vi "mod_Create Continuous MSK.vi"(0 "PN Sequence Order":i32, 1 "MSK System Parameters":T2, 3 "TX Filter":T1(ring), 4 "Filter Length":i32, 5 "error in (no error)":errorcluster, 6 "Symbol Rate, Hz":dbl format="%.2f", 7 "Alpha":dbl format="%.2f") -> (14 "output complex waveform":T3 {"Y" format="%.3f"; "dt" format="%^.2e"; "t0" format="%.4f"}, 17 "samples per symbol":i32, 19 "error out":errorcluster)   [LabVIEW 2020, in "niDMT.lvlib"]
uses:
  <vilib>/addons/Modulation/niDMT.lvlib
  <vilib>/addons/Modulation/Analog/controls/Complex Data Waveform.ctl
  <vilib>/addons/Modulation/Digital/Support/Controls/MSK System Parameters.ctl
  <vilib>/addons/Modulation/Digital/General/MT Generate Bits (Galois, PN Order).vi
  <vilib>/addons/Modulation/Analog/support/mod_Set Error Source.vi
  <vilib>/addons/Modulation/Digital/Support/Common/Validators/mod_Generate Bits Validate.vi
  <vilib>/addons/Modulation/Digital/Support/Common/Validators/mod_Generate Filter Coefficients Validate.vi
  <vilib>/addons/Modulation/Digital/General/subVIs/mod_Generate Filter Coefficients.vi
  <vilib>/addons/Modulation/Digital/General/subVIs/mod_Generate Bits PN Sequence.vi
  <vilib>/addons/Modulation/niAMT.lvlib
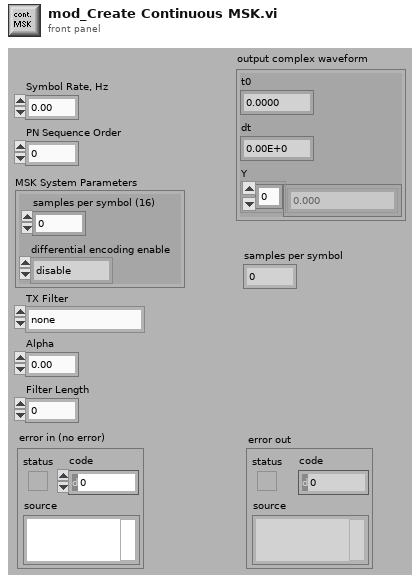
[diagram p1: front panel]
types:
  T1 = enum16{"none", "Raised Cosine", "Root Raised Cos", "Gaussian"}
  T2 = typedef "niDMT.lvlib/MSK System Parameters.ctl" = cluster{"differential encoding enable":enum16{"disable", "enable"}, "samples per symbol (16)":i32}
  T3 = typedef "niAMT.lvlib/Complex Data Waveform.ctl" = cluster{"t0":dbl, "dt":dbl, "Y":cdb[]}
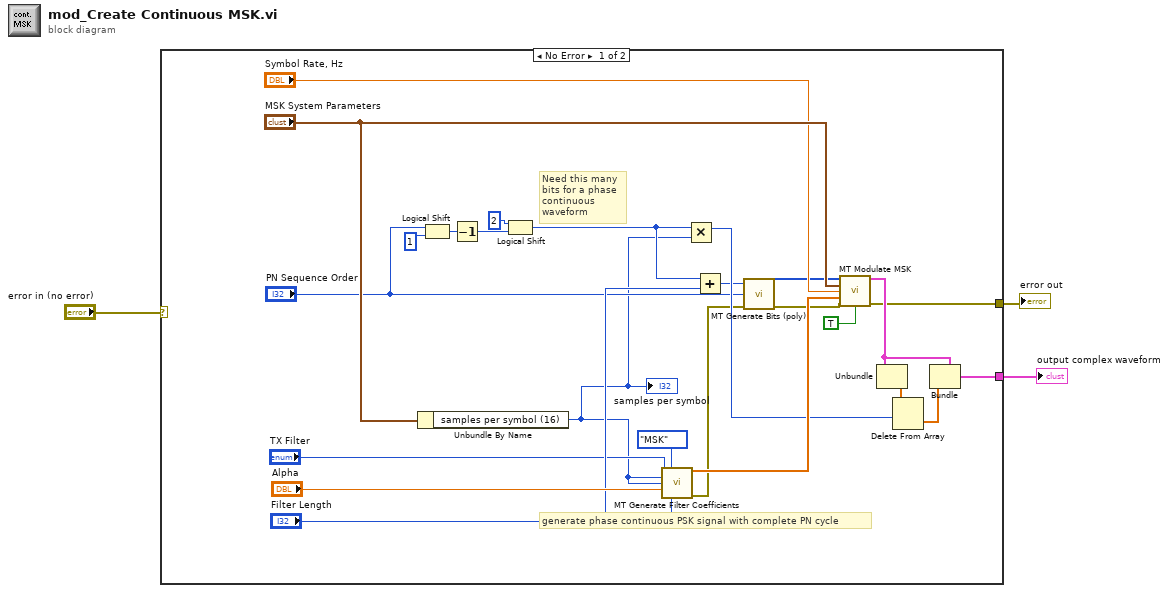
[diagram p0: block diagram]
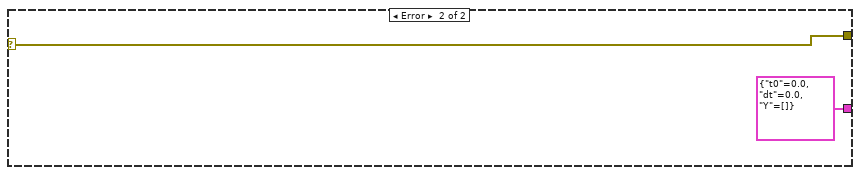
[diagram p2: hidden frame]
diagram:
  n1 = case shown="No Error" "error in (no error)" {
    selector: "error in (no error)" -> [_ w30]
    tunnel: [w28 cluster{"t0":dbl, "dt":dbl, "Y":cdb[]} {"t0"=0.0, "dt"=0.0, "Y"=[]} ("output complex waveform")] -> w3
    tunnel: [w5 w30] -> w2
    frame No Error {
      # "Need this many bits for a phase continuous waveform"
      # "generate phase continuous PSK signal with complete PN cycle"
      n2 = Unbundle By Name("MSK System Parameters") -> ("samples per symbol (16)"=w4:i32)
      "samples per symbol" <- w4
      n3 = Logical Shift(y="PN Sequence Order", x=1) -> (x << y=w10:i32)
      n4 = Decrement(x=w10) -> (x-1=w26:i32)
      n5 = Logical Shift(y=2, x=w26) -> (x << y=w25:i32)
      n6 = call <vilib>:"MT Generate Filter Coefficients.vi"("pulse shaping filter (none)"="TX Filter", "modulation type"=enum16{"FSK", "PSK", "QAM", "MSK"}."MSK" ("Modulation Type"), "pulse shaping samples per symbol (16)"=w4, "matched samples per symbol (16)"=w4, "filter parameter"="Alpha", "filter length (symbols)"="Filter Length") -> ("pulse shaping filter coefficients"=w18:dbl[], "error out"=w7:errorcluster)  [unwired: 1 in, 7 out]
      n7 = Multiply(x=w25, y=w4) -> (x*y=w16:i32)
      n8 = Add(x=w25, y="Filter Length") -> (x+y=w12:i32)
      n9 = call-poly <vilib>:"MT Generate Bits (poly).vi"("total bits (128)"=w12, "PN sequence order (9)"="PN Sequence Order", "error in (no error)"=w7) -> ("output bit stream"=w17:i8[], "error out"=w6:errorcluster)  [unwired: 2 in, 9 out]
      n10 = call <vilib>:"MT Modulate MSK.vi"("input bit stream"=w17, "MSK system parameters"="MSK System Parameters", "symbol rate (Hz)"="Symbol Rate, Hz", "pulse shaping filter coefficients"=w18, "error in (no error)"=w6, "reset? (T)"=TRUE ("Reset (T)")) -> ("output complex waveform"=w20:T3, "error out"=w5:errorcluster)  [unwired: 1 in, 7 out]
      n11 = Unbundle(w20) -> ("Y"=w13:cdb[])  [unwired: 2 out]
      n12 = Delete From Array(array=w13, length=w16) -> (deleted portion=w14:cdb[])  [unwired: 1 in, 1 out]
      n13 = Bundle(cluster=w20, "Y"=w14) -> (w28:T3)  [unwired: 2 out]
    }
    frame Error {
    }
  }
  "output complex waveform" <- w3
  "error out" <- w2
